vi "Datalogger.vi"() -> ()   [LabVIEW 2021]
panel:
  in  "stop":bool
  out "Database Connection":refnum<k7>
  out "String":string
  out "Time Stamp":timestamp
  out "Waveform Chart":i32(graph)
  out "Logging interval":dbl=100.0
  out "error out":errorcluster
  in  "error in (no error)":errorcluster
  in  "Settings":bool
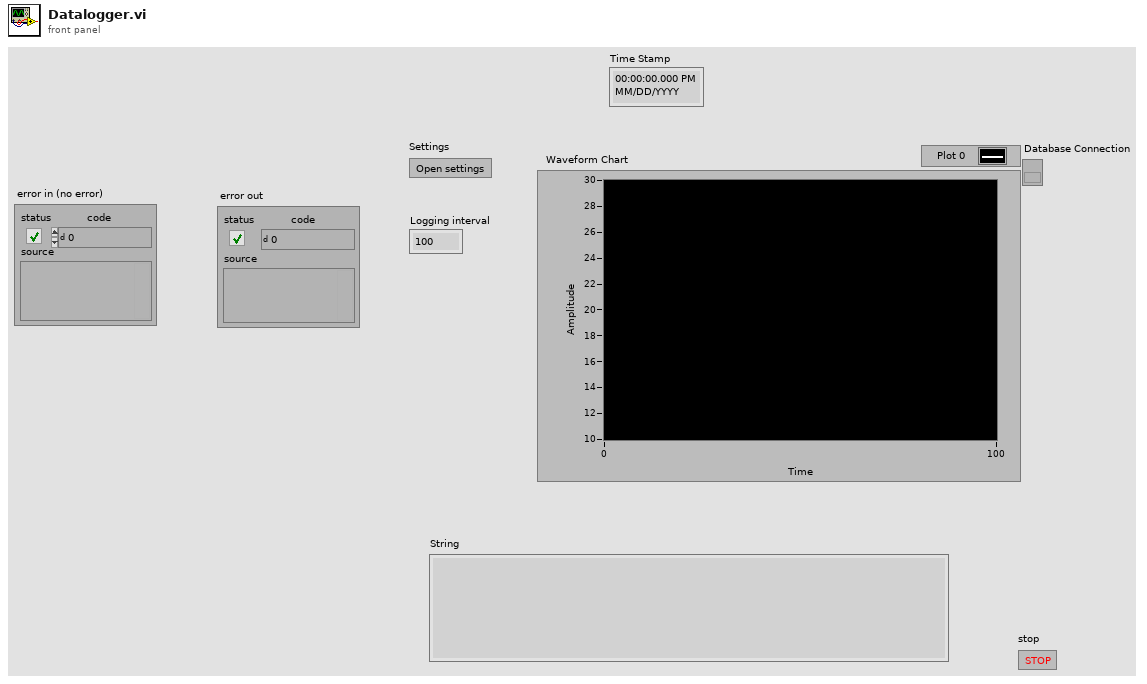
[diagram p1: front panel]
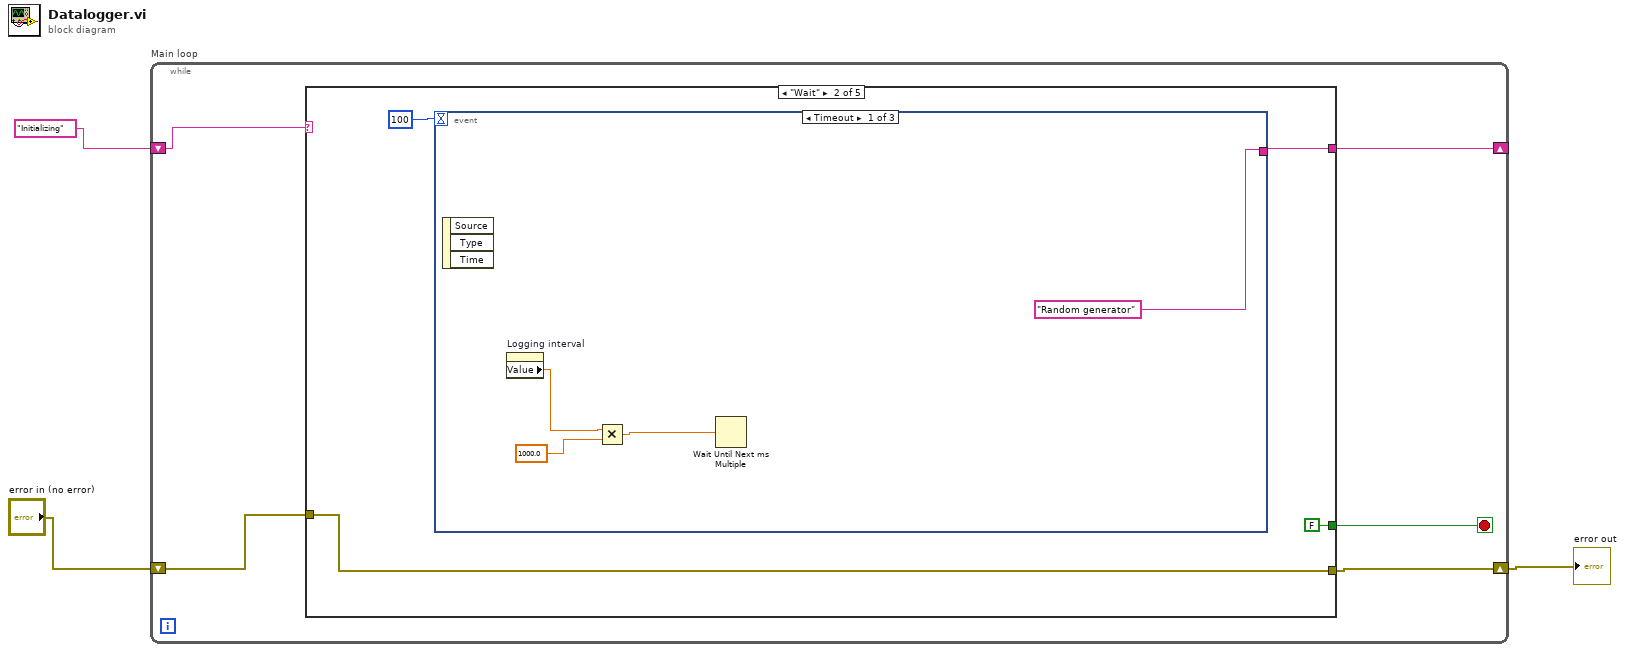
[diagram p0: block diagram]
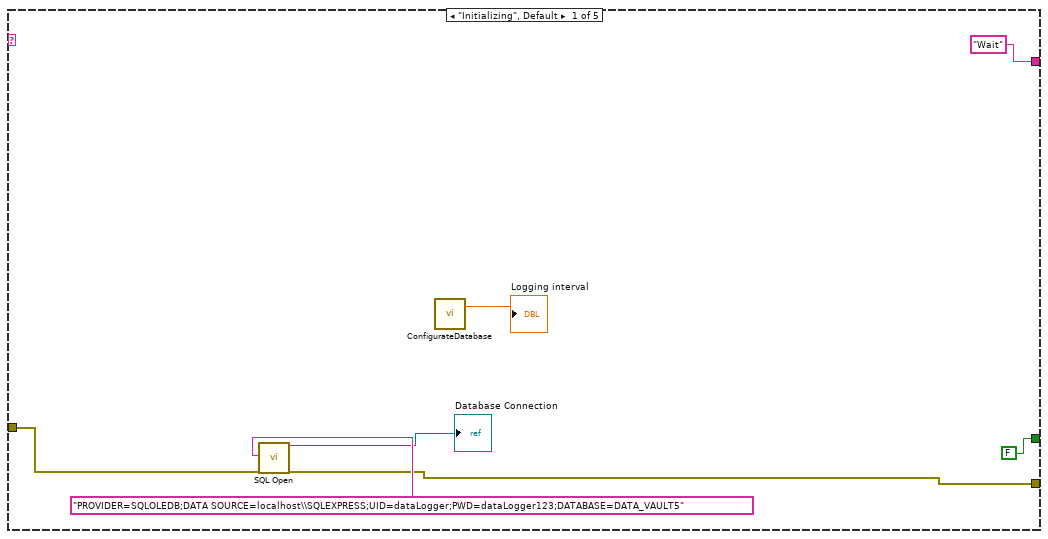
[diagram p2: hidden frame]
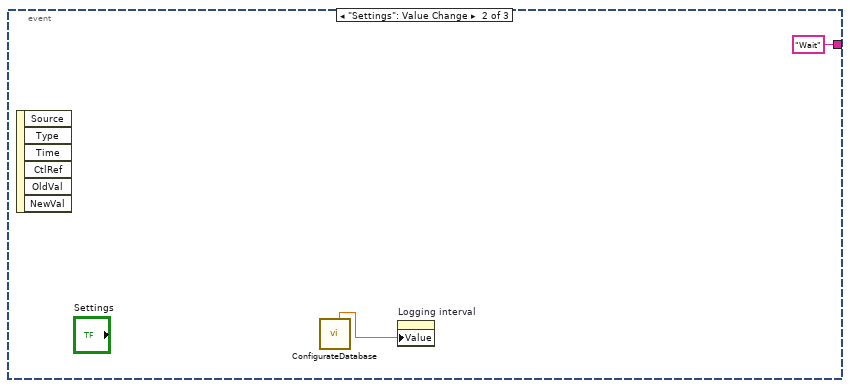
[diagram p3: hidden frame]
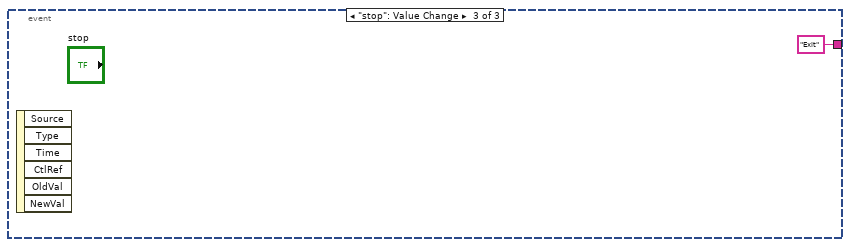
[diagram p4: hidden frame]
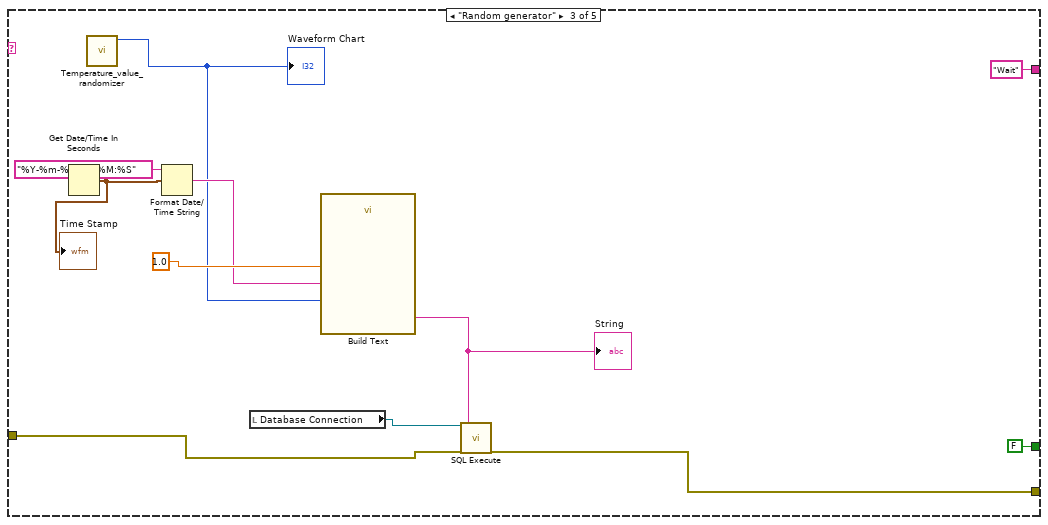
[diagram p5: hidden frame]
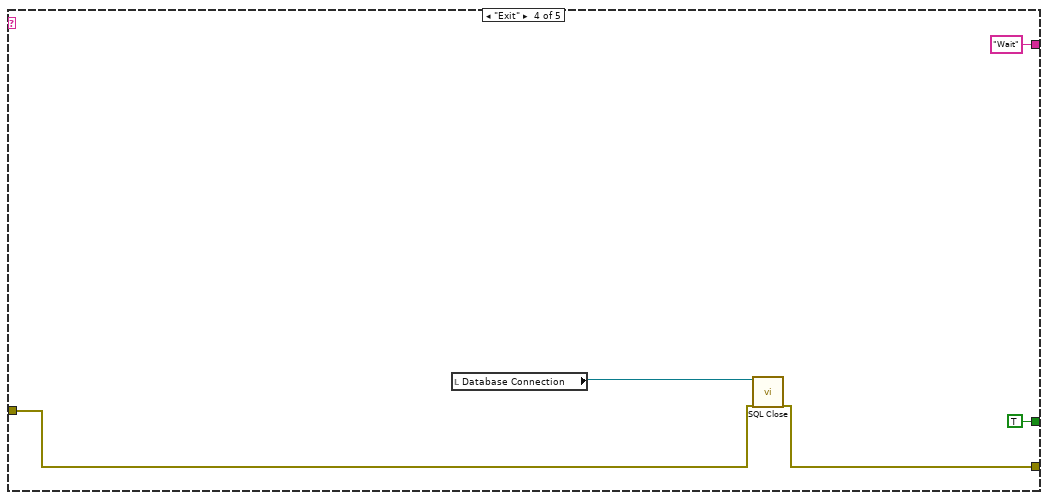
[diagram p6: hidden frame]
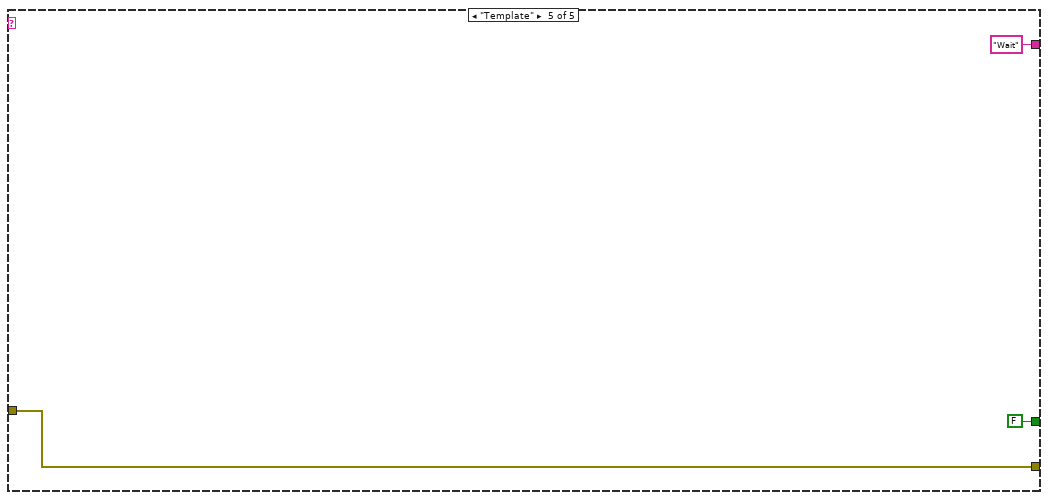
[diagram p7: hidden frame]
diagram:
  n1 = while "Main loop" {
    shift-right: [w7] -> _
    shift-left: "Initializing" -> [w8]
    shift-right: [w4] -> w1
    shift-left: "error in (no error)" -> [w5]
    stop <- w6 stop-if-true
    n2 = case shown="\"Wait\"" w8 {
      tunnel: ["Wait" w17 "Wait" "Wait" "Wait"] -> w7
      tunnel: [FALSE FALSE FALSE TRUE FALSE] -> w6
      tunnel: w5 -> [w10 w16 w29 w39 w43]
      tunnel: [w9 w16 w27 w38 w43] -> w4
      frame "Initializing", Default {
        n3 = call <vilib>:"SQL Open.vi"("ConnectionString In"="PROVIDER=SQLOLEDB;DATA SOURCE=localhost\\SQLEXPRESS;UID=dataLogger;PWD=dataLogger123;DATABASE=DATA_VAULT5", "Error in (no error)"=w10) -> ("Connection Out"=→"Database Connection":refnum<k7>, "Error out"=w9:errorcluster)  [unwired: 16 in]
        n4 = call "ConfigurateDatabase.vi"() -> ("Logging interval"=→"Logging interval":dbl)  [unwired: 11 in]
      }
      frame "Wait" {
        n5 = event shown="[0] Timeout" {
          selector: _ -> [_ _ _]
          dyn-events: _ -> [_ _ _]
          timeout: 100 -> [_ _ _]
          tunnel: ["Random generator" "Wait" "Exit"] -> w17
          event Timeout {
            n6 = event-data() -> ()  [unwired: 1 in, 3 out]
            n7 = property on="Logging interval" class="DigNum (strict)"() -> ("Value"=w20:dbl)  [unwired: 2 in, 2 out]
            n8 = Multiply(x=w20, y=1000.0) -> (x*y=w21:dbl)
            n9 = Wait Until Next ms Multiple(millisecond multiple=w21) -> ()  [unwired: 1 out]
          }
          event "Settings": Value Change {
            n10 = event-data() -> ()  [unwired: 1 in, 6 out]
            n11 = call "ConfigurateDatabase.vi"() -> ("Logging interval"=w25:dbl)  [unwired: 11 in]
            n12 = property on="Logging interval" class="DigNum (strict)"("Value"=w25) -> ()  [unwired: 2 in, 2 out]
          }
          event "stop": Value Change {
            n13 = event-data() -> ()  [unwired: 1 in, 6 out]
          }
        }
      }
      frame "Random generator" {
        n14 = Get Date/Time In Seconds() -> (seconds since 1Jan1904=w34:timestamp)
        "Time Stamp" <- w34
        n15 = call "Temperature_value_randomizer.vi"() -> ("Temperature Value"=w32:i32)  [unwired: 11 in]
        "Waveform Chart" <- w32
        n16 = Format Date/Time String(time format string (%c)="%Y-%m-%d %H:%M:%S", seconds (now)=w34) -> (date/time string=w33:string)  [unwired: 1 in]
        n17 = local read "Database Connection"() -> (w28:refnum<k7>)
        n18 = call "Build Text"("tag_id"=1.0, "timestamp"=w33, "measurement_value"=w32) -> ("Result"=w30:string)  [unwired: 11 in, 1 out]
        "String" <- w30
        n19 = call <vilib>:"SQL Execute.vi"("Connection In"=w28, "SQL Query"=w30, "Error in (no error)"=w29) -> ("Error out"=w27:errorcluster)  [unwired: 15 in, 1 out]
      }
      frame "Exit" {
        n20 = local read "Database Connection"() -> (w40:refnum<k7>)
        n21 = call <vilib>:"SQL Close.vi"("Connection In"=w40, "Error in (no error)"=w39) -> ("Error out"=w38:errorcluster)  [unwired: 17 in]
      }
      frame "Template" {
      }
    }
  }
  "error out" <- w1
